vi "Read.vi"   [LabVIEW 2015, in "Stanford Research 830.lvlib"]
doc: "Reads data in several methods."
uses:
  <instrlib>/Stanford Research 830/Stanford Research 830.lvlib
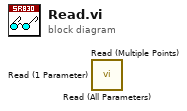
[diagram p0: block diagram]
diagram:
  n1 = call <instrlib>:"Read (All Parameters).vi"() -> ()  [unwired: 9 in, 3 out]
  n2 = call <instrlib>:"Read (Multiple Points).vi"() -> ()  [unwired: 9 in, 3 out]
  n3 = call <instrlib>:"Read (1 Parameter).vi"() -> ()  [unwired: 9 in, 3 out]
